vi "fpga_8ch_Timestamping_BaselineCh.vi"(2 "Signal IN":T1, 3 "Baseline Ch":u8, 4 "Scheduler":u8, 5 "Main clock":u32) -> (0 "Timestamp bundle":T2, 1 "Data available":T1)   [LabVIEW 2011]
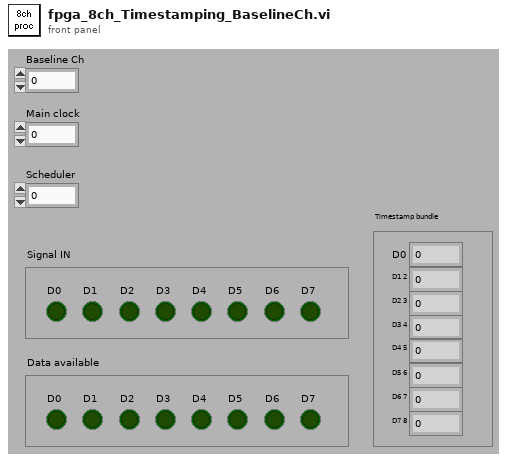
[diagram p1: front panel]
types:
  T1 = cluster{"D0":bool, "D1":bool, "D2":bool, "D3":bool, "D4":bool, "D5":bool, "D6":bool, "D7":bool}
  T2 = cluster{"D0":u32, "D1 2":u32, "D2 3":u32, "D3 4":u32, "D4 5":u32, "D5 6":u32, "D6 7":u32, "D7 8":u32}
  T3 = cluster{"Data Available":bool, "Data Available":bool, "Data Available":bool, "Data Available":bool, "Data Available":bool, "Data Available":bool, "Data Available":bool, "Data Available":bool}
  T4 = cluster{"32 bit Output":u32, "32 bit Output":u32, "32 bit Output":u32, "32 bit Output":u32, "32 bit Output":u32, "32 bit Output":u32, "32 bit Output":u32, "32 bit Output":u32}
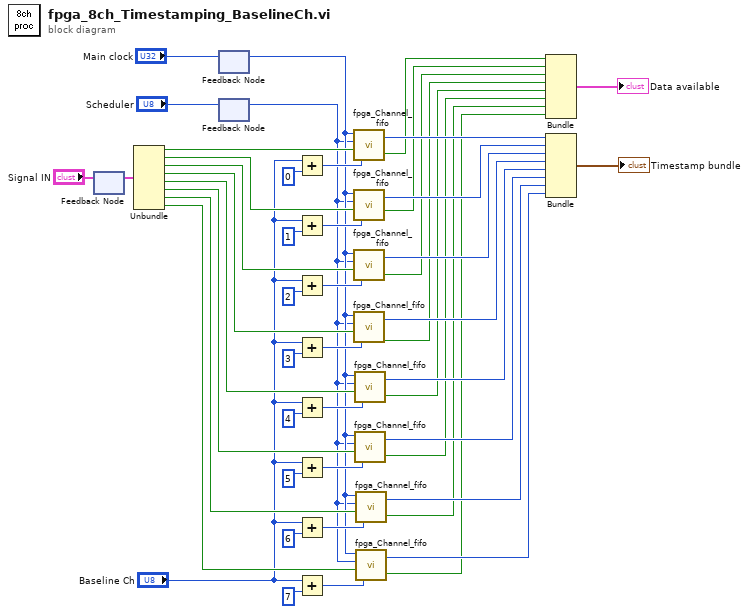
[diagram p0: block diagram]
diagram:
  n1 = feedback-in #1("Signal IN") -> ()
  n2 = feedback #1() -> (w1:T1)  [unwired: 1 in]
  n3 = Unbundle(w1) -> ("D0"=w48:bool, "D1"=w47:bool, "D2"=w46:bool, "D3"=w45:bool, "D4"=w44:bool, "D5"=w43:bool, "D6"=w42:bool, "D7"=w41:bool)
  n4 = feedback-in #2("Main clock") -> ()
  n5 = feedback #2() -> (w4:u32)  [unwired: 1 in]
  n6 = feedback #3() -> (w2:u8)  [unwired: 1 in]
  n7 = feedback-in #3("Scheduler") -> ()
  n8 = Add(x="Baseline Ch", y=u8 0 ("ID")) -> (x+y=w21:u8)
  n9 = Add(x="Baseline Ch", y=u8 1 ("ID")) -> (x+y=w8:u8)
  n10 = Add(x="Baseline Ch", y=u8 2 ("ID")) -> (x+y=w9:u8)
  n11 = Add(x="Baseline Ch", y=u8 3 ("ID")) -> (x+y=w6:u8)
  n12 = Add(x="Baseline Ch", y=u8 4 ("ID")) -> (x+y=w10:u8)
  n13 = Add(x="Baseline Ch", y=u8 5 ("ID")) -> (x+y=w11:u8)
  n14 = Add(x="Baseline Ch", y=u8 6 ("ID")) -> (x+y=w12:u8)
  n15 = Add(x="Baseline Ch", y=u8 7 ("ID")) -> (x+y=w13:u8)
  n16 = call "fpga_Channel_fifo.vi"("ID"=w21, "Signal IN"=w48, "Schedule"=w2, "Main clock"=w4) -> ("Data Available"=w31:bool, "32 bit Output"=w40:u32)
  n17 = call "fpga_Channel_fifo.vi"("ID"=w8, "Signal IN"=w47, "Schedule"=w2, "Main clock"=w4) -> ("Data Available"=w30:bool, "32 bit Output"=w39:u32)
  n18 = call "fpga_Channel_fifo.vi"("ID"=w9, "Signal IN"=w46, "Schedule"=w2, "Main clock"=w4) -> ("Data Available"=w29:bool, "32 bit Output"=w38:u32)
  n19 = call "fpga_Channel_fifo.vi"("ID"=w6, "Signal IN"=w45, "Schedule"=w2, "Main clock"=w4) -> ("Data Available"=w28:bool, "32 bit Output"=w37:u32)
  n20 = call "fpga_Channel_fifo.vi"("ID"=w10, "Signal IN"=w44, "Schedule"=w2, "Main clock"=w4) -> ("Data Available"=w27:bool, "32 bit Output"=w36:u32)
  n21 = call "fpga_Channel_fifo.vi"("ID"=w11, "Signal IN"=w43, "Schedule"=w2, "Main clock"=w4) -> ("Data Available"=w26:bool, "32 bit Output"=w35:u32)
  n22 = call "fpga_Channel_fifo.vi"("ID"=w12, "Signal IN"=w42, "Schedule"=w2, "Main clock"=w4) -> ("Data Available"=w25:bool, "32 bit Output"=w34:u32)
  n23 = call "fpga_Channel_fifo.vi"("ID"=w13, "Signal IN"=w41, "Schedule"=w2, "Main clock"=w4) -> ("Data Available"=w24:bool, "32 bit Output"=w33:u32)
  n24 = Bundle("Data Available"=w31, "Data Available"=w30, "Data Available"=w29, "Data Available"=w28, "Data Available"=w27, "Data Available"=w26, "Data Available"=w25, "Data Available"=w24) -> (→"Data available":T3)  [unwired: 1 in]
  n25 = Bundle("32 bit Output"=w40, "32 bit Output"=w39, "32 bit Output"=w38, "32 bit Output"=w37, "32 bit Output"=w36, "32 bit Output"=w35, "32 bit Output"=w34, "32 bit Output"=w33) -> (→"Timestamp bundle":T4)  [unwired: 1 in]
